vi "Labels Load.vi"(8 "error in (no error)":errorcluster, 11 "Labels":T2) -> (0 "error out":errorcluster, 3 "File Open Reference out":T1)   [LabVIEW 2018]
panel:
  # "LOAD LABELs"
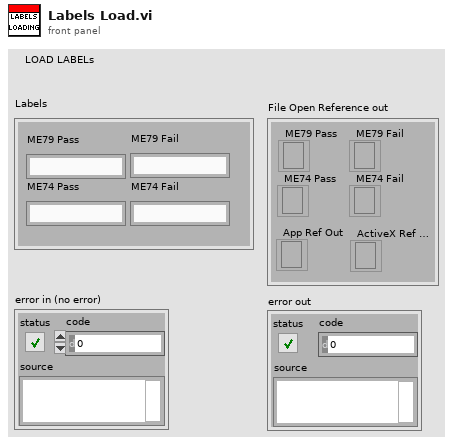
[diagram p1: front panel]
types:
  T1 = cluster{"ME79 Pass":refnum<k7>, "ME79 Fail":refnum<k7>, "ME74 Pass":refnum<k7>, "ME74 Fail":refnum<k7>, "App Ref Out":refnum<k7>, "ActiveX Ref Out":refnum<k7>}
  T2 = cluster{"ME79 Pass":string, "ME79 Fail":string, "ME74 Pass":string, "ME74 Fail":string}
  T3 = cluster{"Open":refnum<k7>, "Open":refnum<k7>, "Open":refnum<k7>, "Open":refnum<k7>, "Formats":refnum<k7>, "BarTender.IBtApplication":refnum<k7>}
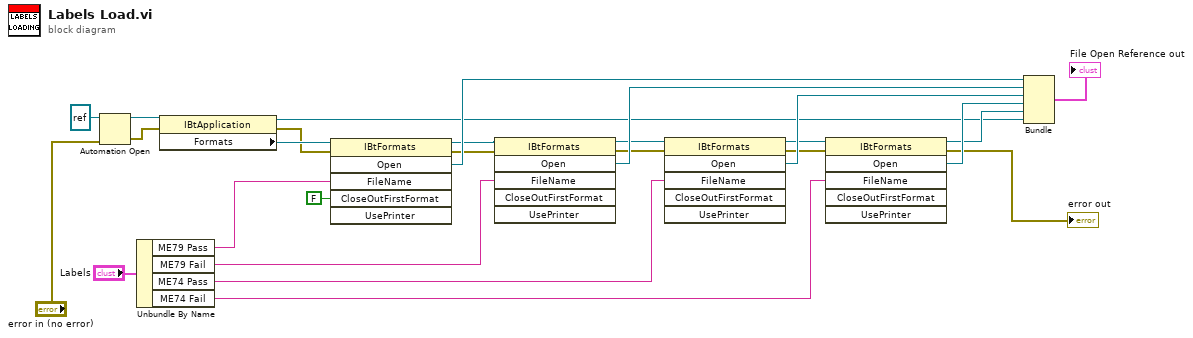
[diagram p0: block diagram]
diagram:
  n1 = Automation Open(error in (no error)="error in (no error)", Automation Refnum=refnum<k7> refnum ("BarTender.IBtApplication")) -> (Automation Refnum=w25:refnum<k7>, error out=w1:errorcluster)  [unwired: 2 in]
  n2 = Unbundle By Name("Labels") -> ("ME79 Pass"=w22:string, "ME79 Fail"=w21:string, "ME74 Pass"=w20:string, "ME74 Fail"=w19:string)
  n3 = property class="IBtApplication"(reference=w25, error in=w1) -> (reference out=w3:refnum<k7>, error out=w9:errorcluster, "Formats"=w23:refnum<k7>)
  n4 = invoke class="IBtFormats" method="Open"(reference=w23, error in=w9, "FileName"=w22, "CloseOutFirstFormat"=FALSE) -> (reference out=w12:refnum<k7>, error out=w8:errorcluster, "Open"=w17:refnum<k7>)  [unwired: 2 in, 3 out]
  n5 = invoke class="IBtFormats" method="Open"(reference=w12, error in=w8, "FileName"=w21) -> (reference out=w11:refnum<k7>, error out=w7:errorcluster, "Open"=w16:refnum<k7>)  [unwired: 3 in, 3 out]
  n6 = invoke class="IBtFormats" method="Open"(reference=w11, error in=w7, "FileName"=w20) -> (reference out=w10:refnum<k7>, error out=w6:errorcluster, "Open"=w15:refnum<k7>)  [unwired: 3 in, 3 out]
  n7 = invoke class="IBtFormats" method="Open"(reference=w10, error in=w6, "FileName"=w19) -> (reference out=w4:refnum<k7>, error out=→"error out":errorcluster, "Open"=w14:refnum<k7>)  [unwired: 3 in, 3 out]
  n8 = Bundle("Open"=w17, "Open"=w16, "Open"=w15, "Open"=w14, "Formats"=w4, "BarTender.IBtApplication"=w3) -> (→"File Open Reference out":T3)  [unwired: 1 in]
